vi "leedlet.vi"(11 "NXT/EV3":T1) -> (3 "NXT/EV3 out":T1)   [LabVIEW 2014, in "Janga.lvrbt"]
uses:
  Janga.lvrbt
  <vilib>/NXT/Subs/LVHSConnector.ctl
  <vilib>/NXT/LegoClasses/BrickReference/BrickReference.lvclass
  <vilib>/NXT/Remote Library/Sound/NXT_SoundVolume.ctl
  <vilib>/NXT/Dual Mode Library/Sound/PlaySoundFile.vi
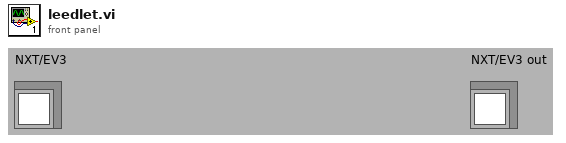
[diagram p1: front panel]
types:
  T1 = typedef "LVHSConnector.ctl" = refnum<class "BrickReference.lvclass">
  T2 = typedef "NXT_SoundVolume.ctl" = u8
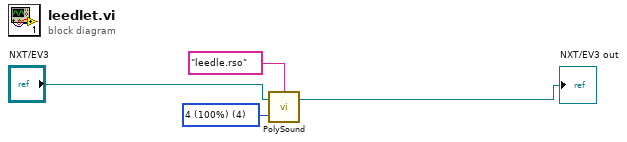
[diagram p0: block diagram]
diagram:
  w3 = T2 4 items=["0 (Mute)", "1 (25%)", "2 (50%)", "3 (75%)", "4 (100%)"] ("Volume (4)")
  n1 = call-poly <vilib>:"PolySound.vi"("Volume (4)"=w3, "NXT/EV3"="NXT/EV3", "Filename (*.rso/*.rsf)"="leedle.rso") -> ("NXT/EV3"=→"NXT/EV3 out":T1)  [unwired: 1 in]
